vi "Decode Transducer Data.vi"(9 "Vref":dbl, 11 "Transducer Value":u16[](array[numeric])) -> (2 "TD Data":T1[](array[typedef]) {"Value" scale=0.0..10.0})   [LabVIEW 2015]
uses:
  Transducer Calibration Display.ctl
  Sensor Enum.ctl
  Sensor Port Mapping Global Action.ctl
  Transducer Calibration Global Action.ctl
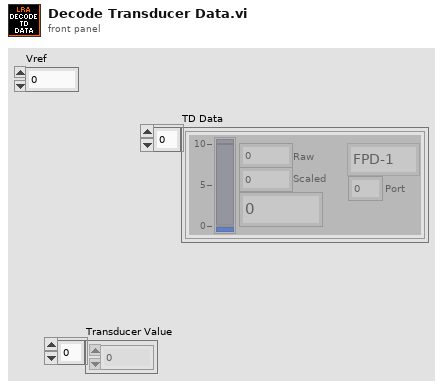
[diagram p1: front panel]
types:
  T1 = typedef "Transducer Calibration Display.ctl" = cluster{"Value":dbl, "Raw":dbl, "Scaled":dbl, "Sensor Name":T2, "Port":u32}
  T2 = typedef "Sensor Enum.ctl" = enum16{"FPD-1", "FPD-2", "FPD-3", "OPD-1", "OPD-2", "OPD-3", "AP-1", "VBAT", "VCOMP", "ICOMP", "TD10"}
  T3 = typedef "Sensor Port Mapping Global Action.ctl" = enum16{"Get", "Set"}
  T4 = typedef "Sensor Port Mapping.ctl" = cluster{"Sensor":T2, "Thermocouple?":bool, "Port":u32}
  T5 = typedef "Transducer Calibration Global Action.ctl" = enum16{"Get", "Set"}
  T6 = typedef "Transducer Calibration Control.ctl" = cluster{"Scale":dbl, "Offset":dbl}
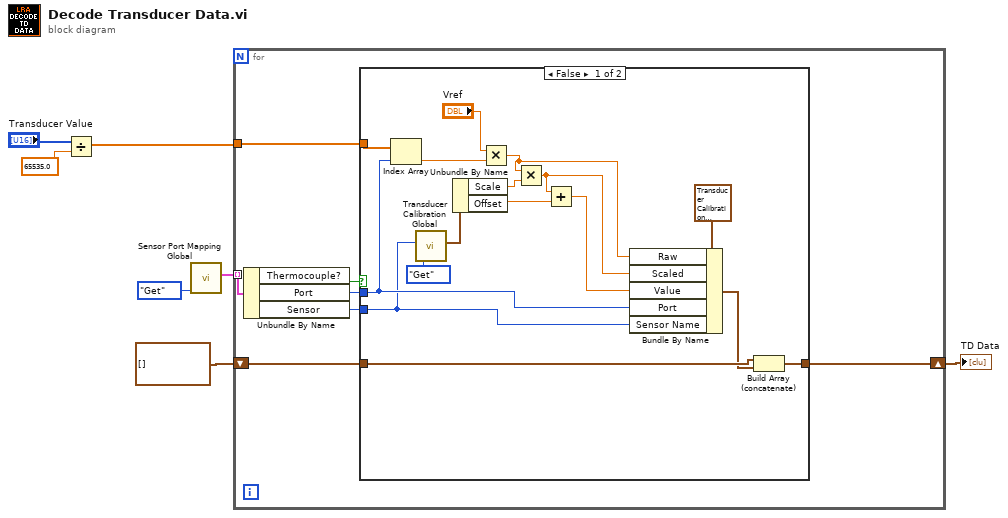
[diagram p0: block diagram]
diagram:
  n1 = Divide(x="Transducer Value", y=65535.0) -> (x/y=w3:dbl[])
  n2 = call "Sensor Port Mapping Global.vi"("Action"=Sensor_Port_Mapping_Global_Action."Get") -> ("Mapping List"=w4:T4[])  [unwired: 10 in]
  n3 = for {
    tunnel: w4 -> [w14] mode=indexing
    tunnel: w3 -> [w10]
    shift-right: [w8] -> w1
    shift-left: T1[] [] -> [w9]
    n4 = Unbundle By Name(w14) -> ("Thermocouple?"=w13:bool, "Port"=w12:u32, "Sensor"=w11:T2)
    n5 = case shown="False" w13 {
      tunnel: w12 -> [w26 _]
      tunnel: w11 -> [w20 _]
      tunnel: w10 -> [w29 _]
      tunnel: w9 -> [w19 w31]
      tunnel: [w28 w31] -> w8
      frame False {
        n6 = Index Array(array=w29, index=w26) -> (element=w17:dbl)
        n7 = call "Transducer Calibration Global.vi"("Action"=Transducer_Calibration_Global_Action."Get", "Sensor"=w20) -> ("Calibration Data"=w25:T6)  [unwired: 9 in]
        n8 = Unbundle By Name(w25) -> ("Scale"=w24:dbl, "Offset"=w22:dbl)
        n9 = Multiply(x="Vref", y=w17) -> (x*y=w15:dbl)
        n10 = Multiply(x=w15, y=w24) -> (x*y=w23:dbl)
        n11 = Add(x=w23, y=w22) -> (x+y=w21:dbl)
        n12 = Bundle By Name(cluster=T1 {"Value"=6.829268292682927, "Raw"=0.0, "Scaled"=0.0, "Sensor Name"=enum."FPD-1", "Port"=0} ("Cluster 3"), "Raw"=w15, "Scaled"=w23, "Value"=w21, "Port"=w26, "Sensor Name"=w20) -> (w18:T1)
        n13 = Build Array (concatenate)(w19, w18) -> (w28:T1[])
      }
      frame True {
      }
    }
  }
  "TD Data" <- w1
